vi "Set_Tree.vi"(8 "error in (no error)":errorcluster, 10 "ctl":refnum<vi>, 11 "IB_Tree in":refnum<class "IB_Tree.lvclass">) -> (0 "error out":errorcluster, 3 "IB_Tree out":refnum<class "IB_Tree.lvclass">)   [LabVIEW 2020, in "IB_Tree.lvclass"]
uses:
  <vilib>/AppBuilder/IB_Classes/Tree/IB_Tree.lvclass
  <vilib>/AppBuilder/IB_Classes/Tree/IB_Tree.lvclass/IB_Tree.ctl
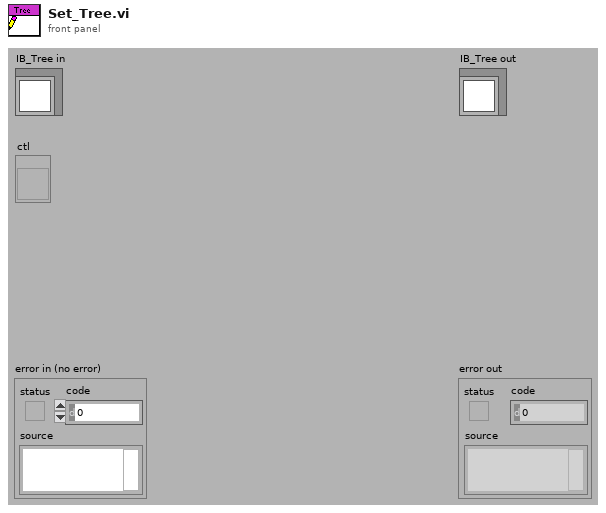
[diagram p1: front panel]
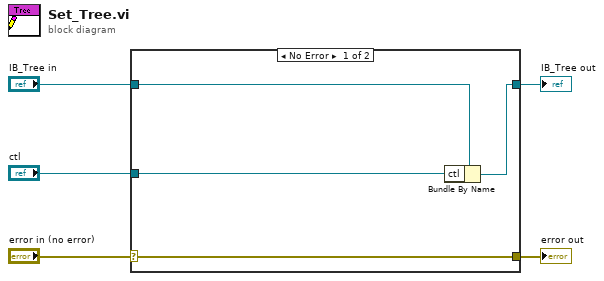
[diagram p0: block diagram]
diagram:
  n1 = case shown="No Error" "error in (no error)" {
    selector: "error in (no error)" -> [w9 w10]
    tunnel: [w9 w10] -> w4
    tunnel: [w7 w11] -> w2
    tunnel: "IB_Tree in" -> [w8 w11]
    tunnel: "ctl" -> [w6 _]
    frame No Error {
      n2 = Bundle By Name(cluster=w8, "ctl"=w6) -> (w7:refnum<class "IB_Tree.lvclass">)
    }
    frame Error {
    }
  }
  "error out" <- w4
  "IB_Tree out" <- w2
